vi "Indicate Tubes.vi"(8 "error in (no error)":errorcluster, 11 "Storage in":refnum<class "Storage.lvclass">) -> (0 "error out":errorcluster, 3 "Storage out":refnum<class "Storage.lvclass">)   [LabVIEW 2015, in "AMS UI.lvlib" / "Storage.lvclass"]
uses:
  Storage.lvclass
  Storage.lvclass/Storage.ctl
  subs/Sample/Sample.lvclass/Sample.ctl
  subs/Sample/Sample.lvclass
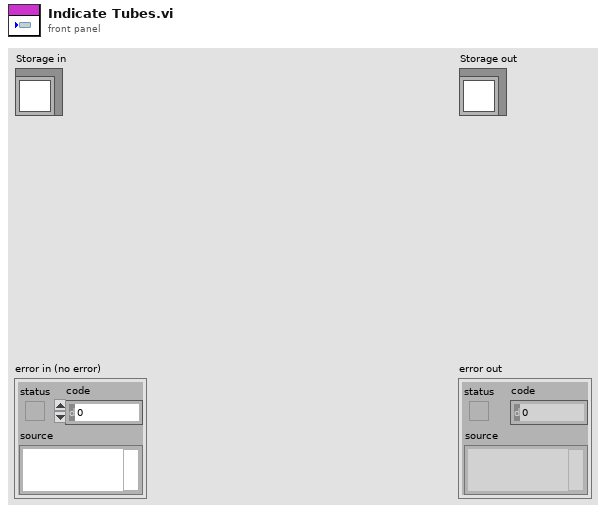
[diagram p1: front panel]
types:
  T1 = typedef "Sample Container.ctl" = cluster{"Sample In":refnum<k21>, "Sample Name":refnum<k21>, "Ti Cathode":refnum<k21>, "SampleQ":refnum<queue>}
  T2 = typedef "FP Control Refs Cluster.ctl" = cluster{"Liquid N Valve References":T3, "Main Line Valve Refs":T4, "Transfer Line Container":refnum<vi>, "Storage Containers":refnum<vi>[], "Sample Refs":T5, "Syringe Ctrl Refs ":T6, "Baratrons Chart":refnum<vi>, "Capillary Container":refnum<vi>, "Preparation Container":refnum<vi>, "Monkey Mode":refnum<vi>}
  T3 = typedef "Liquid N Valve Ref Cluster.ctl" = cluster{"Cold Bath H2O HV 100":refnum<vi>, "Cold Bath Cleaning HV 101":refnum<vi>, "Cold Bath Storage 1 HV 102":refnum<vi>, "Cold Bath Storage 2 HV 103":refnum<vi>, "Cold Bath Storage 3 HV 104":refnum<vi>, "Cold Bath Storage 4 HV 105":refnum<vi>, "Cold Bath Syringe HV 106":refnum<vi>, "Liquid N Master Valve HV 107":refnum<vi>}
  T4 = typedef "Main Line Valve Ref Cluster.ctl" = cluster{"Turbo Valve DV313":refnum<vi>, "Prep Line Valve 0 DV300":refnum<vi>, "Storage Valves":refnum<vi>[]}
  T5 = typedef "Sample Valve Refs.ctl" = cluster{"Valves":cluster{"Sample 5 DV318":refnum<vi>, "Sample 4 DV317":refnum<vi>, "Sample 3 DV316":refnum<vi>, "Sample 2 DV315":refnum<vi>, "Sample 1 DV314":refnum<vi>}, "Lines":cluster{"Sample 1":refnum<vi>, "Sample 2":refnum<vi>, "Sample 3":refnum<vi>, "Sample 4":refnum<vi>, "Sample 5":refnum<vi>}}
  T6 = typedef "Syringe Ctrl Refs.ctl" = cluster{"Syringe Home":refnum<vi>, "Syringe Freeze":refnum<vi>, "Syringe TC":refnum<vi>, "Syringe Container":refnum<vi>}
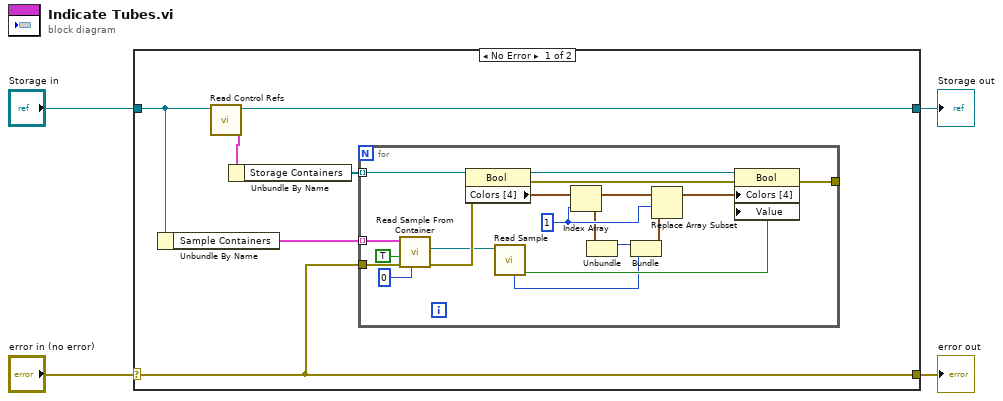
[diagram p0: block diagram]
diagram:
  n1 = case shown="No Error" "error in (no error)" {
    selector: "error in (no error)" -> [w5 w30]
    tunnel: [w5 w30] -> w3
    tunnel: [w8 w29] -> w1
    tunnel: "Storage in" -> [w7 w29]
    frame No Error {
      n2 = Unbundle By Name(w7) -> ("Sample Containers"=w6:T1[])
      n3 = call-dynamic "Read Control Refs.vi"("AMS Gas Actor in"=w7) -> ("Control Refs"=w10:T2, "AMS Gas Actor out"=w8:refnum<class "Storage.lvclass">)  [unwired: 9 in]
      n4 = Unbundle By Name(w10) -> ("Storage Containers"=w9:refnum<vi>[])
      n5 = for {
        tunnel: w9 -> [w28] mode=indexing
        tunnel: [w25] -> _
        tunnel: w6 -> [w18] mode=indexing
        tunnel: w5 -> [w16]
        w23 = 1 ("index")
        n6 = call "Read Sample From Container.vi"("Queue timeout in ms (-1)"=0, "error in (no error)"=w16, "Read from SHV (F)"=TRUE, "Container"=w18) -> ("error out"=w17:errorcluster, "Sample out"=w15:refnum<class "Sample.lvclass">)  [unwired: 3 in, 3 out]
        n7 = property class="Bool"(reference=w28, error in=w17) -> (reference out=w27:refnum<vi>, error out=w26:errorcluster, "Colors [4]"=w24:cluster{u32, u32}[])
        n8 = call "Read Sample.vi"("Sample in"=w15) -> ("Sample In"=w14:bool, "Color"=w13:u32)  [unwired: 6 in, 3 out]
        n9 = Index Array(array=w24, index=w23) -> (element=w19:cluster{u32, u32})
        n10 = Unbundle(w19) -> (w20:u32)  [unwired: 1 out]
        n11 = Bundle(w20, "Color"=w13) -> (w22:cluster{u32, "Color":u32})  [unwired: 1 in]
        n12 = Replace Array Subset(array=w24, new element=w22, index=w23) -> (w21:cluster{u32, u32}[])
        n13 = property class="Bool"(reference=w27, error in=w26, "Colors [4]"=w21, "Value"=w14) -> (error out=w25:errorcluster)  [unwired: 1 out]
      }
    }
    frame Error {
    }
  }
  "error out" <- w3
  "Storage out" <- w1
